vi "Acceleration Move Test.vi"() -> ()   [LabVIEW 2019]
uses:
  <vilib>/rvi/interface/nirviMethod/nirviMethod.xnode
  <vilib>/FPGAPlugInAG/Dynamic/niLvFpga_Abort_Dynamic.vi
  <vilib>/FPGAPlugInAG/Dynamic/niLvFpga_Run_Dynamic.vi
  <vilib>/rvi/interface/nirviReadWriteControl/nirviReadWriteControl.xnode
  NiFpgaLv.dll
  <vilib>/Utility/error.llb/Error Cluster From Error Code.vi
  <vilib>/rvi/interface/Simulation/niFpgaSimulationCallBeginRW.vi
  <vilib>/rvi/errors/niLvFpgaAdjustHostInterfaceError.vi
  <vilib>/platform/TimedLoop/XDataNode/XDataNode.xnode
  <vilib>/Platform/TimedLoop/XDataNode/timing_clust.ctl
  <vilib>/Platform/TimedLoop/XDataNode/XDNodeRunTimeDep.lvlib
  <vilib>/Platform/TimedLoop/XDataNode/wakeup.ctl
  <vilib>/Platform/TimedLoop/XDataNode/nitl_modes.ctl
  <vilib>/rvi/interface/nirviOpenFPGA/nirviOpenFPGA.xnode
  <vilib>/Analysis/NI_AALPro.lvlib
  <vilib>/Instr/_visa.llb/VISA Configure Serial Port (Instr).vi
panel:
  out "實際角度Chart":cluster{"X":dbl, "Y":dbl}(graph)={"X"=-3.299667554384925, "Y"=3.520332445615068} caption="Waveform Chart - dark"
  out "實際角度":cluster{"X":dbl, "Y":dbl, "AccZ":dbl}
  out "Gyro Acceleration Graph":cluster{i32[], "Ideal Acc":dbl[]}[](graph)
  in  "VISA resource name":refnum<visa-resource-name>="COM2"
  out "陀螺儀推算軸長L3":dbl
  out "陀螺儀推算軸長L2":dbl
  out "陀螺儀推算軸長L1":dbl
  out "Axis 3 Real Acceleration Graph":cluster{i32[], "Ideal Acc":dbl[]}[](graph)
  out "Axis 2 Real Acceleration Graph":cluster{i32[], "Ideal Acc":dbl[]}[](graph)
  out "Axis 3 Real Velocity Graph":cluster{i32[], "Ideal Velocity":dbl[]}[](graph)
  out "Axis 2 Real Velocity Graph":cluster{i32[], "Ideal Velocity":dbl[]}[](graph)
  out "Axis 1 Real Acceleration Graph":cluster{i32[], "dX/dt":dbl[]}[](graph)
  out "Axis 1 Real Velocity Graph":cluster{i32[], "Ideal Velocity":dbl[]}[](graph)
  out "Axis 1":cluster{i32[], "Ideal Move":dbl[]}[](graph)
  out "Axis 3":cluster{i32[], "Ideal Move":dbl[]}[](graph)
  out "Axis 2":cluster{i32[], "Ideal Move":dbl[]}[](graph)
  in  "Period":i64=10
  in  "stop":bool
  out "time loop error":errorcluster
  out "Axis 1 速率 (1mm/s)":dbl
  out "Real Period":u32
  out "沖壓":bool
  out "結束了":bool
  out "Voltage\nOutput":dbl
  out "Voltage\nOutput 2":dbl
  out "Voltage\nOutput 3":dbl
  out "Axis 2 速率 (1mm/s)":dbl
  out "Axis 3 速率 (1mm/s)":dbl
  out "shutdown error":errorcluster
  in  "Tab Control":enum32{"Axis Control"}(tab)
  in  "Axis 1~3 Servo on?":bool
  out "Axis 3 Backward Limit":bool
  out "Axis 3 Backward Limit 2":bool
  out "Axis 2 Backward Limit":bool
  out "Axis 2 Backward Limit 2":bool
  in  "Axis 3 Alarm Reset":bool
  in  "Axis 2 Alarm Reset":bool
  in  "Axis 3 Position Reset":bool
  in  "Axis 2 Position Reset":bool
  in  "Axis 1 Alarm Reset":bool
  in  "Axis 1 Position Reset":bool
  in  "Axis 3 Speed":fxp<+/-,64,32>
  in  "Axis 2 Speed":fxp<+/-,64,32>
  out "Axis 3 Encoder Position (Counts)":i32
  out "Axis 2 Encoder Position (Counts)":i32
  out "Axis 1 Encoder Position (Counts)":i32
  in  "Axis 1 Spped":fxp<+/-,64,32>
  in  "Axis 2 Servo on?":bool
  in  "Axis 3 Servo on?":bool
  in  "Axis 1 Servo on?":bool
  out "Axis 1 Forward Limit":bool
  out "Axis 1 Backward Limit":bool
  out "Timed Out?":bool
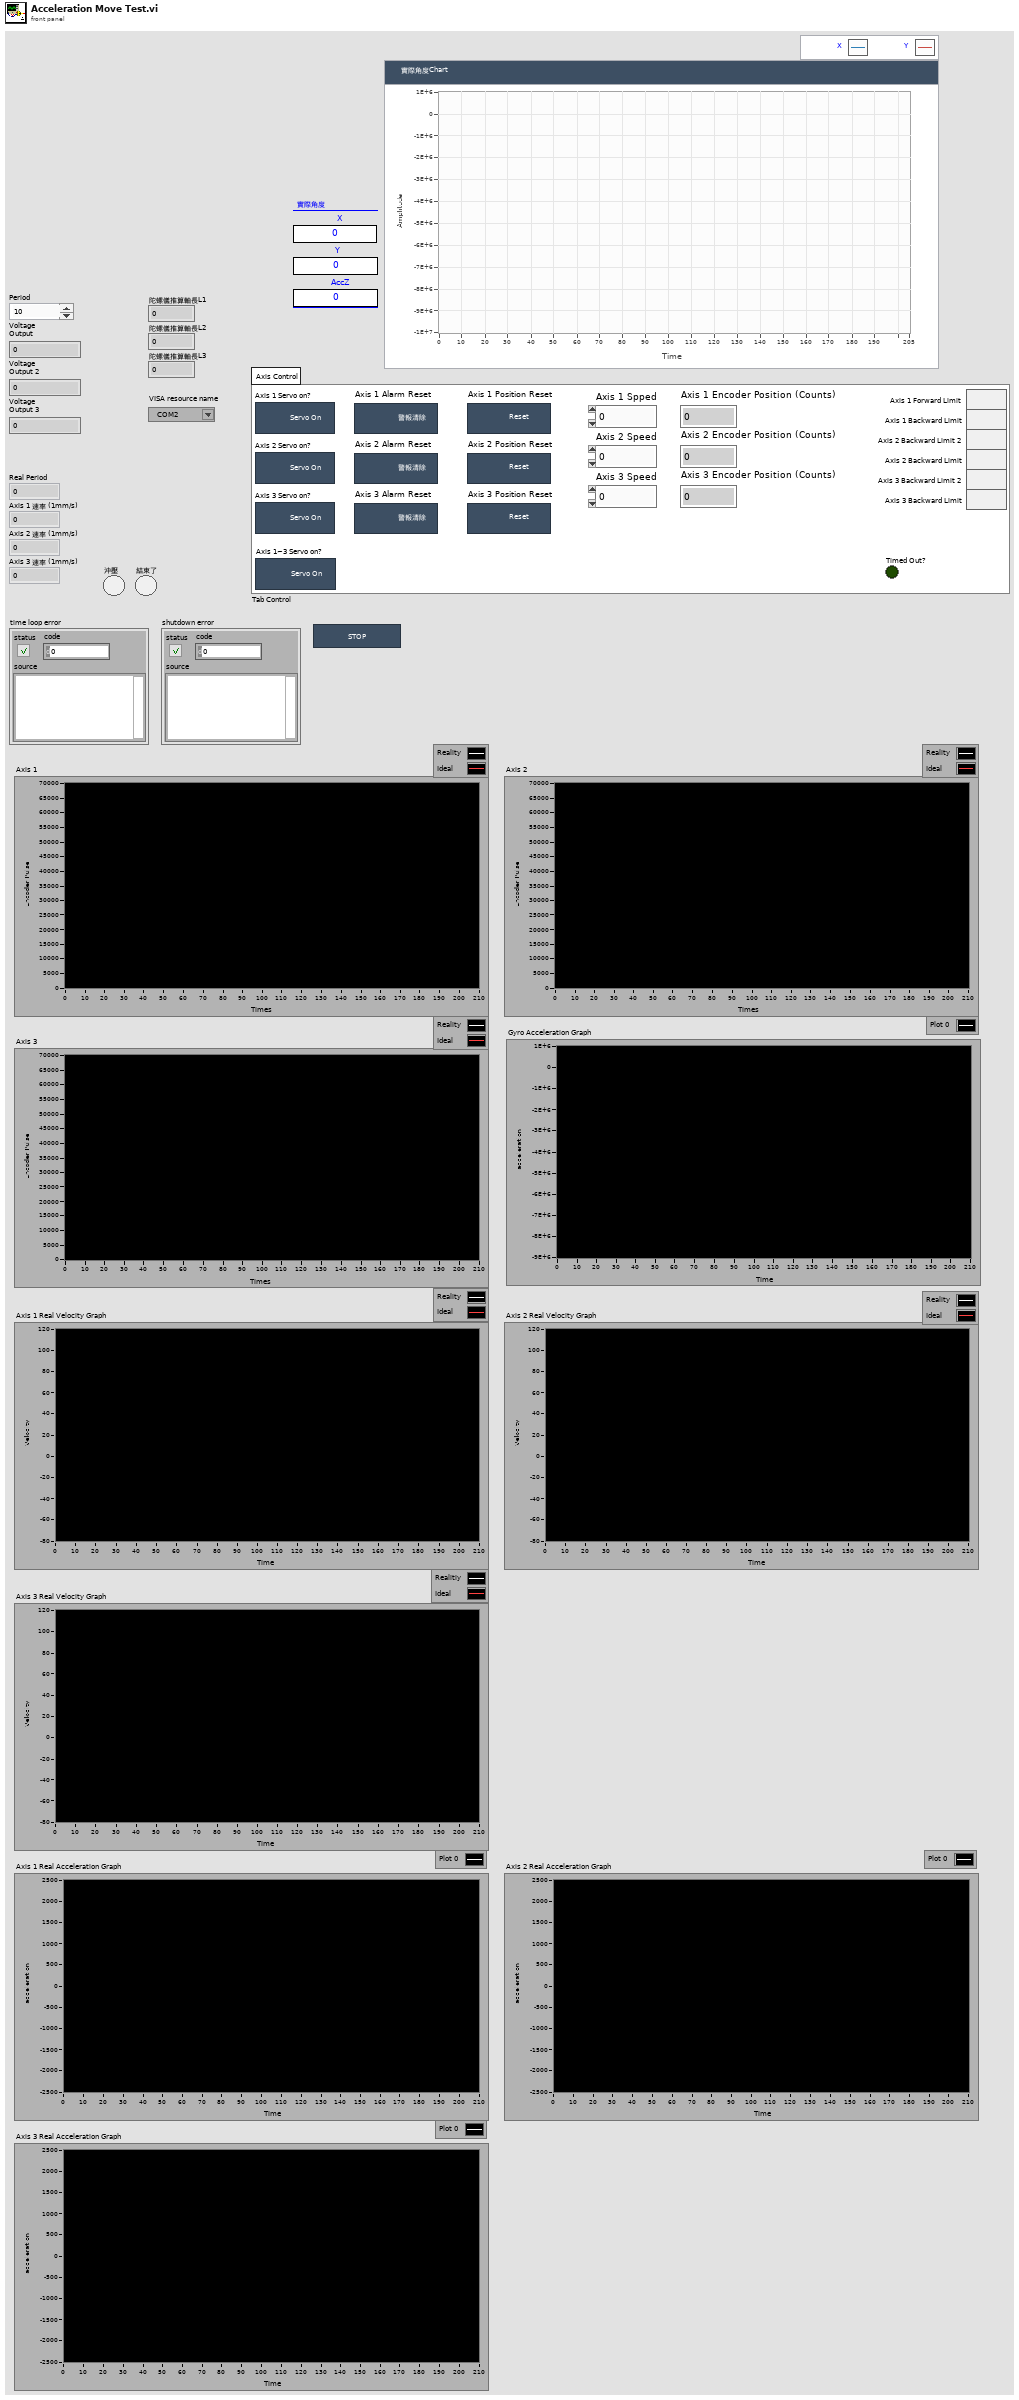
[diagram p1: front panel]
types:
  T1 = enum16{"open", "replace", "create", "open or create", "replace or create", "replace or create with confirmation"}
  T2 = cluster{"Acceleration 1":dbl, "Acceleration 2":dbl, "Acceleration 3":dbl, "Acceleration 4":dbl, "Acceleration 5":dbl, "Acceleration 6":dbl, "Acceleration 7":dbl, "Acceleration 8":dbl}
  T3 = cluster{"Time 1":dbl, "Time 2":dbl, "Time 3":dbl, "Time 4":dbl, "Time 5":dbl, "Time 6":dbl, "Time 7":dbl, "Time 8":dbl}
  T4 = typedef "XDNodeRunTimeDep.lvlib/timing_clust.ctl" = cluster{"Expected End [f-1]":u64, "Actual End [f-1]":u64, "Finished Late? [f-1]":bool, "Expected End [i-1]":u64, "Actual End [i-1]":u64, "Finished Late? [i-1]":bool, "Expected Start [i]":u64, "Actual Start [i]":u64, "Expected Start [f]":u64, "Actual Start [f]":u64, "Source Name":string, "Structure Name":string, "Period":i64, "Deadline":i64, "Offset":i64, "Start":i64, "Priority":i32, "Timeout":i32, "Mode":T5, "Wakeup Reason":T6, "Error":errorcluster, "Source Type":string, "Secondary Source Type":string, "Global End Time":u64, "Global Start Time":u64, "Frame Duration":u64, "Iteration Duration":u64, "Assigned CPU":i32, "I/O Scan Engine Mode":u32}
  T5 = typedef "XDNodeRunTimeDep.lvlib/nitl_modes.ctl" = enum32{"No Change", "Process missed periods, maintain original phase", "Discard missed periods, maintain original phase", "Process missed periods, ignore original phase", "Discard missed periods, ignore original phase"}
  T6 = typedef "XDNodeRunTimeDep.lvlib/wakeup.ctl" = enum32{"Normal", "Aborted", "Asynchronous wakeup", "Timing source error", "Timed loop error", "Timeout"}
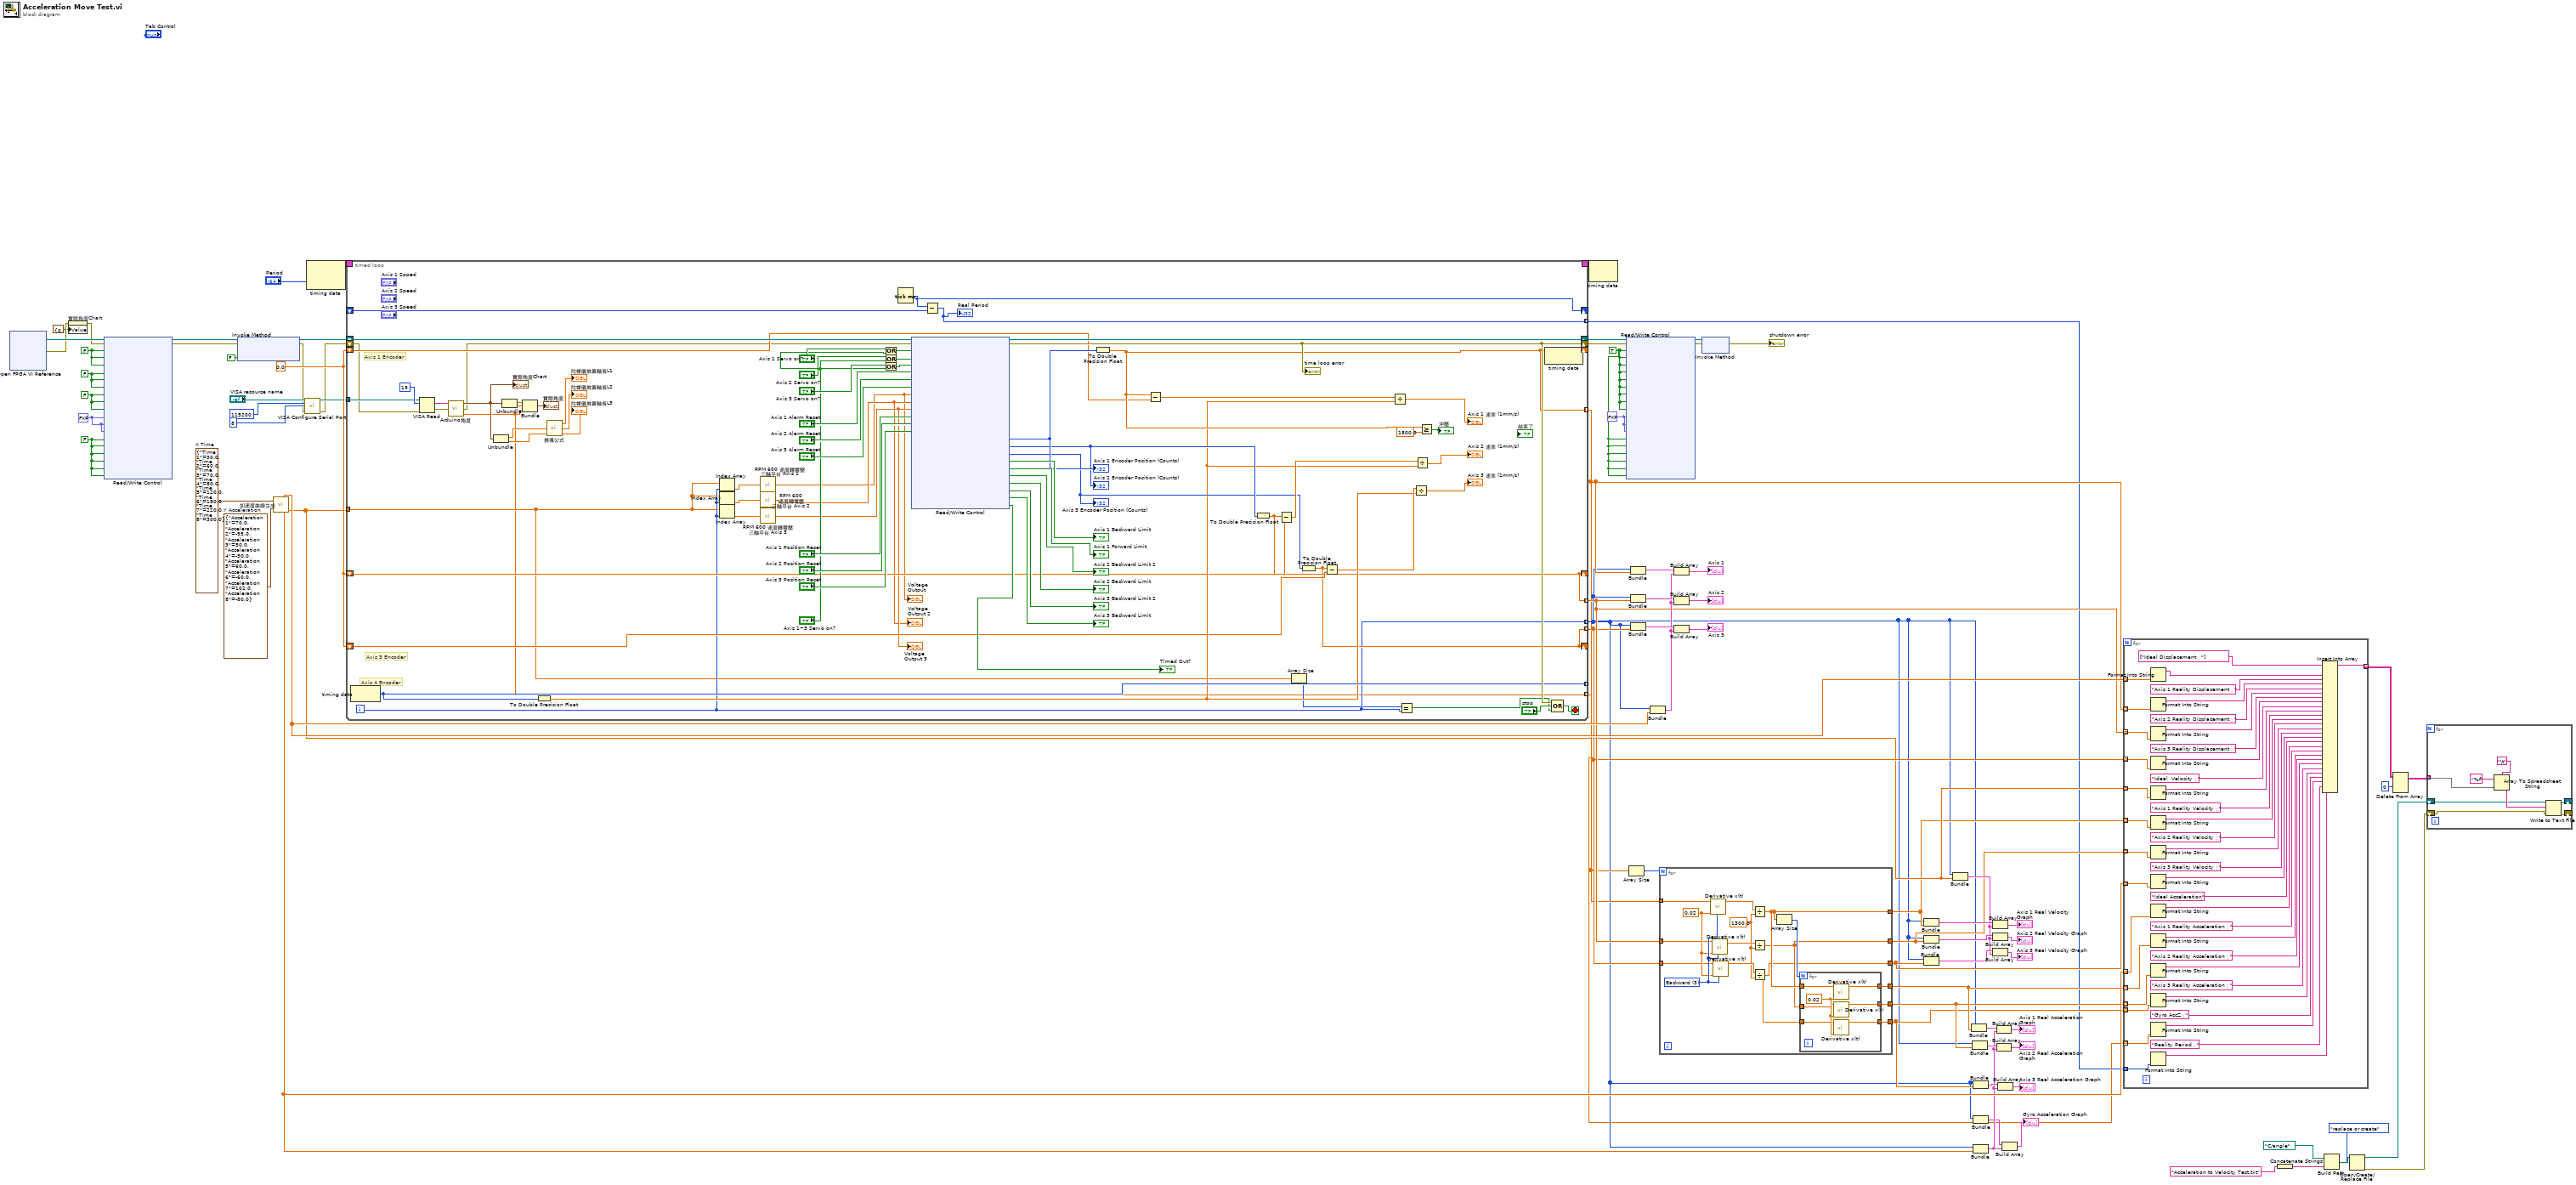
[diagram p0: block diagram]
diagram:
  w58 = T2 {"Acceleration 1"=70.0, "Acceleration 2"=-95.0, "Acceleration 3"=50.0, "Acceleration 4"=-50.0, "Acceleration 5"=60.0, "Acceleration 6"=-60.0, "Acceleration 7"=102.0, "Acceleration 8"=-80.0}  # Y Acceleration
  w60 = T3 {"Time 1"=30.0, "Time 2"=60.0, "Time 3"=70.0, "Time 4"=80.0, "Time 5"=120.0, "Time 6"=180.0, "Time 7"=220.0, "Time 8"=300.0}  # X Time
  w62 = FALSE
  w64 = FALSE
  w70 = 0.0
  w68 = fxp<+,1,1> 0.0
  w67 = TRUE
  w65 = FALSE
  w63 = fxp<+,1,1> 0.0
  w66 = FALSE
  n1 = xnode "Open FPGA VI Reference"() -> ("FPGA VI Reference Out"=w61:refnum<k20>, "error out"=w3:errorcluster)  [unwired: 2 in]
  n2 = property on="實際角度Chart" class="WFChart (strict)"(error in=w3, "Value"=cluster{"X":dbl, "Y":dbl} {"X"=0.0, "Y"=0.0} ("實際角度Chart")) -> (error out=w2:errorcluster)  [unwired: 1 in, 1 out]
  n3 = xnode "Read/Write Control"("FPGA VI Reference In"=w61, "error in"=w2, "Axis 1 Servo on?"=w66, "Axis 2 Servo on?"=w66, "Axis 3 Servo on?"=w66, "Axis 1 Alarm Reset"=w65, "Axis 2 Alarm Reset"=w65, "Axis 3 Alarm Reset"=w65, "Axis 1 Position Reset"=w64, "Axis 2 Position Reset"=w64, "Axis 3 Position Reset"=w64, "Axis 1 Voltage In"=w63, "Axis 2 Voltage In"=w63, "Axis 3 Voltage In"=w63, "Axis 1 Backward Limit"=w62, "Axis 1 Forward Limit"=w62, "Axis 2 Forward Limit"=w62, "Axis 2 Backward Limit"=w62, "Axis 3 ForWard Limit"=w62, "Axis 3 Backward Limit"=w62) -> ("FPGA VI Reference Out"=w79:refnum<k20>, "error out"=w78:errorcluster)
  n4 = xnode "Invoke Method"("FPGA VI Reference In"=w79, "error in"=w78, "Wait Until Done (F)"=FALSE) -> ("FPGA VI Reference Out"=w76:refnum<k20>, "error out"=w10:errorcluster)
  n5 = call "加速度曲線生成.vi"("X Time"=w60, "Y Velocity"=w58) -> ("Ideal Move"=w36:dbl[], "Ideal Acc"=w19:dbl[], "Ideal Velocity"=w32:dbl[])  [unwired: 3 out]
  n6 = call-poly "VISA Configure Serial Port"("VISA resource name"="VISA resource name", "baud rate (9600)"=u32 115200, "data bits (8)"=u16 8, "error in (no error)"=w10) -> ("VISA resource name out"=w11:refnum<visa-resource-name>, "error out"=w9:errorcluster)  [unwired: 10 in]
  n7 = node-c288("Period") -> (w81:T4)  [unwired: 1 in]
  n8 = timed-loop {
    shift-right: [w153] -> w72
    shift-left: w76 -> [w152]
    shift-right: [w120] -> w73
    shift-left: w9 -> [w84]
    timing: w81 -> [_]
    timing-out: [_] -> w80
    shift-right: [w115] -> _
    shift-left: w70 -> [w114]
    tunnel: [w119] -> _ mode=indexing
    shift-right: [w149] -> _
    shift-left: _ -> [w150]
    tunnel: [w109] -> w15 mode=indexing
    shift-right: [w108] -> _
    shift-left: w70 -> [w111]
    shift-right: [w107] -> _
    shift-left: w70 -> [w112]
    tunnel: [w106] -> w7 mode=indexing
    tunnel: [w115] -> w33 mode=indexing
    tunnel: [w108] -> w35 mode=indexing
    tunnel: [w107] -> w34 mode=indexing
    tunnel: w32 -> [w98]
    tunnel: w11 -> [w85]
    tunnel: [w82] -> w4 mode=indexing
    i -> [w106]
    stop <- w151 stop-if-true
    # "Axis 3 Encoder"
    # "Axis 4 Encoder"
    # "Axis 1 Encoder"
    n9 = node-c288() -> (w119:i64)  [unwired: 1 in]
    n10 = VISA Read(VISA resource name=w85, byte count=u32 19, error in (no error)=w84) -> (read buffer=w88:string, error out=w87:errorcluster)  [unwired: 2 out]
    n11 = call "Arduino角度.vi"("error in"=w87, "read buffer"=w88) -> ("AccZ"=w82:dbl, "error out"=w83:errorcluster, "Waveform Chart"=w94:cluster{dbl, dbl})  [unwired: 1 in]
    "實際角度Chart" <- w94
    n12 = Unbundle(w94) -> (w92:dbl, w93:dbl)
    n13 = Unbundle(w94) -> (w95:dbl, w96:dbl)
    n14 = Bundle(w95, w96, "AccZ"=w82) -> (→"實際角度":cluster{dbl, dbl, "AccZ":dbl})  [unwired: 1 in]
    n15 = To Double Precision Float(number=w119) -> (double precision float=w113:dbl)
    n16 = call "推導公式.vi"("be"=w93, "al"=w92) -> ("L3"=→"陀螺儀推算軸長L3":dbl, "L2"=→"陀螺儀推算軸長L2":dbl, "L1"=→"陀螺儀推算軸長L1":dbl)  [unwired: 1 in]
    n17 = Index Array(array=w98, index=w106) -> (element=w103:dbl)
    n18 = Index Array(array=w98, index=w106) -> (element=w102:dbl)
    n19 = Index Array(array=w98, index=w106) -> (element=w104:dbl)
    n20 = call "RPM 600 速度轉電壓 三軸平台 Axis 1.vi"("Speed (1mm/s)"=w103) -> ("Voltage\nOutput"=w99:dbl)
    "Voltage\nOutput" <- w99
    n21 = call "RPM 600 速度轉電壓 三軸平台 Axis 2.vi"("Speed (1mm/s)"=w102) -> ("Voltage\nOutput"=w100:dbl)
    "Voltage\nOutput 2" <- w100
    n22 = call "RPM 600 速度轉電壓 三軸平台 Axis 3.vi"("Speed (1mm/s)"=w104) -> ("Voltage\nOutput"=w101:dbl)
    "Voltage\nOutput 3" <- w101
    n23 = Or(x="Axis 1 Servo on?", y="Axis 1~3 Servo on?") -> (x .or. y?=w132:bool)
    n24 = Or(x="Axis 2 Servo on?", y="Axis 1~3 Servo on?") -> (x .or. y?=w129:bool)
    n25 = Or(x="Axis 3 Servo on?", y="Axis 1~3 Servo on?") -> (x .or. y?=w127:bool)
    n26 = Tick Count (ms)() -> (millisecond timer value=w149:u32)
    n27 = xnode "Read/Write Control"("FPGA VI Reference In"=w152, "error in"=w83, "Axis 1 Servo on?"=w132, "Axis 2 Servo on?"=w129, "Axis 3 Servo on?"=w127, "Axis 1 Alarm Reset"="Axis 1 Alarm Reset", "Axis 2 Alarm Reset"="Axis 2 Alarm Reset", "Axis 3 Alarm Reset"="Axis 3 Alarm Reset", "Axis 1 Voltage In"=w99, "Axis 2 Voltage In"=w100, "Axis 3 Voltage In"=w101, "Axis 1 Position Reset"="Axis 1 Position Reset", "Axis 2 Position Reset"="Axis 2 Position Reset", "Axis 3 Position Reset"="Axis 3 Position Reset") -> ("FPGA VI Reference Out"=w153:refnum<k20>, "error out"=w120:errorcluster, "Axis 1 Encoder Position (Counts)"=w125:i32, "Axis 2 Encoder Position (Counts)"=w123:i32, "Axis 3 Encoder Position (Counts)"=w122:i32, "Axis 1 Backward Limit"=→"Axis 1 Backward Limit":bool, "Axis 1 Forward Limit"=→"Axis 1 Forward Limit":bool, "Axis 2 Backward Limit"=→"Axis 2 Backward Limit 2":bool, "Axis 2 Forward Limit"=→"Axis 2 Backward Limit":bool, "Axis 3 Backward Limit"=→"Axis 3 Backward Limit 2":bool, "Axis 3 ForWard Limit"=→"Axis 3 Backward Limit":bool, "Timed Out?"=→"Timed Out?":bool)
    "time loop error" <- w120
    "Axis 1 Encoder Position (Counts)" <- w125
    "Axis 2 Encoder Position (Counts)" <- w123
    "Axis 3 Encoder Position (Counts)" <- w122
    n28 = Subtract(x=w149, y=w150) -> (x-y=w109:u32)
    "Real Period" <- w109
    n29 = To Double Precision Float(number=w125) -> (double precision float=w115:dbl)
    n30 = Subtract(x=w115, y=w114) -> (x-y=w154:dbl)
    n31 = To Double Precision Float(number=w123) -> (double precision float=w108:dbl)
    n32 = Subtract(x=w108, y=w111) -> (x-y=w124:dbl)
    n33 = Array Size(array=w98) -> (size(s)=w105:i32)
    n34 = To Double Precision Float(number=w122) -> (double precision float=w107:dbl)
    n35 = Subtract(x=w107, y=w112) -> (x-y=w121:dbl)
    n36 = Divide(x=w154, y=w113) -> (x/y=→"Axis 1 速率 (1mm/s)":dbl)
    n37 = Equal?(x=w105, y=w106) -> (x = y?=w110:bool)
    n38 = Divide(x=w121, y=w113) -> (x/y=→"Axis 3 速率 (1mm/s)":dbl)
    n39 = Divide(x=w124, y=w113) -> (x/y=→"Axis 2 速率 (1mm/s)":dbl)
    n40 = Greater Or Equal?(x=w115, y=1800.0) -> (x >= y?=→"沖壓":bool)
    n41 = node-c288() -> ()  [unwired: 1 in, 1 out]
    n42 = Compound Arithmetic op=OR(w120, "stop", w110) -> (w151:bool)
  }
  n43 = node-c288(w80) -> ()  [unwired: 1 out]
  n44 = xnode "Read/Write Control"("FPGA VI Reference In"=w72, "error in"=w73, "Axis 1 Servo on?"=w67, "Axis 2 Servo on?"=w67, "Axis 3 Servo on?"=w67, "Axis 1 Alarm Reset"=w67, "Axis 2 Alarm Reset"=w67, "Axis 3 Alarm Reset"=w67, "Axis 1 Position Reset"=w67, "Axis 2 Position Reset"=w67, "Axis 3 Position Reset"=w67, "Axis 1 Voltage In"=w68, "Axis 2 Voltage In"=w68, "Axis 3 Voltage In"=w68, "Axis 1 Backward Limit"=w67, "Axis 1 Forward Limit"=w67, "Axis 2 Forward Limit"=w67, "Axis 2 Backward Limit"=w67, "Axis 3 ForWard Limit"=w67, "Axis 3 Backward Limit"=w67) -> ("FPGA VI Reference Out"=w75:refnum<k20>, "error out"=w74:errorcluster)
  n45 = Array Size(array=w33) -> (size(s)=w59:i32)
  n46 = Bundle(w7, w33) -> (w50:cluster{i32[], dbl[]})  [unwired: 1 in]
  n47 = Bundle(w7, w35) -> (w49:cluster{i32[], dbl[]})  [unwired: 1 in]
  n48 = Bundle(w7, w34) -> (w48:cluster{i32[], dbl[]})  [unwired: 1 in]
  n49 = Bundle(w7, "Ideal Move"=w36) -> (w47:cluster{i32[], "Ideal Move":dbl[]})  [unwired: 1 in]
  n50 = for {
    N: w59 -> [_]
    tunnel: w33 -> [w173]
    tunnel: [w171] -> w31
    tunnel: [w169] -> w18
    tunnel: w35 -> [w166]
    tunnel: w34 -> [w165]
    tunnel: [w164] -> w17
    tunnel: [w163] -> w16
    tunnel: [w159] -> w30
    tunnel: [w158] -> w29
    w168 = u16 3 items=["2nd Order Central", "4th Order Central", "Forward", "Backward"] ("method")
    w160 = 1300.0 ("dt")
    w167 = 0.02 ("dt")
    n51 = call <vilib>:"Derivative x(t).vi"("method"=w168, "dt"=w167, "X"=w173) -> ("dX/dt"=w172:dbl[])  [unwired: 7 in, 1 out]
    n52 = call <vilib>:"Derivative x(t).vi"("method"=w168, "dt"=w167, "X"=w166) -> ("dX/dt"=w162:dbl[])  [unwired: 7 in, 1 out]
    n53 = call <vilib>:"Derivative x(t).vi"("method"=w168, "dt"=w167, "X"=w165) -> ("dX/dt"=w161:dbl[])  [unwired: 7 in, 1 out]
    n54 = Divide(x=w172, y=w160) -> (x/y=w171:dbl[])
    n55 = Divide(x=w162, y=w160) -> (x/y=w159:dbl[])
    n56 = Divide(x=w161, y=w160) -> (x/y=w158:dbl[])
    n57 = Array Size(array=w171) -> (size(s)=w170:i32)
    n58 = for {
      N: w170 -> [_]
      tunnel: w171 -> [w179]
      tunnel: [w180] -> w169
      tunnel: w159 -> [w177]
      tunnel: w158 -> [w176]
      tunnel: [w175] -> w164
      tunnel: [w174] -> w163
      w178 = 0.02 ("dt")
      n59 = call <vilib>:"Derivative x(t).vi"("dt"=w178, "X"=w179) -> ("dX/dt"=w180:dbl[])  [unwired: 8 in, 1 out]
      n60 = call <vilib>:"Derivative x(t).vi"("dt"=w178, "X"=w177) -> ("dX/dt"=w175:dbl[])  [unwired: 8 in, 1 out]
      n61 = call <vilib>:"Derivative x(t).vi"("dt"=w178, "X"=w176) -> ("dX/dt"=w174:dbl[])  [unwired: 8 in, 1 out]
    }
  }
  n62 = Build Array(w50, w47) -> (→"Axis 1":cluster{i32[], "Ideal Move":dbl[]}[])
  n63 = Build Array(w49, w47) -> (→"Axis 2":cluster{i32[], "Ideal Move":dbl[]}[])
  n64 = Build Array(w48, w47) -> (→"Axis 3":cluster{i32[], "Ideal Move":dbl[]}[])
  n65 = xnode "Invoke Method"("FPGA VI Reference In"=w75, "error in"=w74) -> ("error out"=→"shutdown error":errorcluster)  [unwired: 1 out]
  n66 = Bundle(w7, w31) -> (w57:cluster{i32[], dbl[]})  [unwired: 1 in]
  n67 = Bundle(w7, w30) -> (w56:cluster{i32[], dbl[]})  [unwired: 1 in]
  n68 = Bundle(w7, w29) -> (w55:cluster{i32[], dbl[]})  [unwired: 1 in]
  n69 = Bundle(w7, "Ideal Velocity"=w32) -> (w51:cluster{i32[], "Ideal Velocity":dbl[]})  [unwired: 1 in]
  n70 = Bundle(w7, "dX/dt"=w18) -> (w24:cluster{i32[], "dX/dt":dbl[]})  [unwired: 1 in]
  n71 = Bundle(w7, "dX/dt"=w17) -> (w23:cluster{i32[], "dX/dt":dbl[]})  [unwired: 1 in]
  n72 = Bundle(w7, "dX/dt"=w16) -> (w22:cluster{i32[], "dX/dt":dbl[]})  [unwired: 1 in]
  n73 = Bundle(w7, "Ideal Acc"=w19) -> (w8:cluster{i32[], "Ideal Acc":dbl[]})  [unwired: 1 in]
  n74 = Bundle(w7, w4) -> (w6:cluster{i32[], dbl[]})  [unwired: 1 in]
  n75 = Build Array(w57, w51) -> (→"Axis 1 Real Velocity Graph":cluster{i32[], "Ideal Velocity":dbl[]}[])
  n76 = Build Array(w56, w51) -> (→"Axis 2 Real Velocity Graph":cluster{i32[], "Ideal Velocity":dbl[]}[])
  n77 = Build Array(w55, w51) -> (→"Axis 3 Real Velocity Graph":cluster{i32[], "Ideal Velocity":dbl[]}[])
  n78 = Build Array(w24, w8) -> (→"Axis 1 Real Acceleration Graph":cluster{i32[], "Ideal Acc":dbl[]}[])
  n79 = Build Array(w23, w8) -> (→"Axis 2 Real Acceleration Graph":cluster{i32[], "Ideal Acc":dbl[]}[])
  n80 = Build Array(w22, w8) -> (→"Axis 3 Real Acceleration Graph":cluster{i32[], "Ideal Acc":dbl[]}[])
  n81 = Build Array(w6, w8) -> (→"Gyro Acceleration Graph":cluster{i32[], "Ideal Acc":dbl[]}[])
  n82 = for {
    tunnel: [w222] -> w28 mode=indexing
    tunnel: w36 -> [w219] mode=indexing
    tunnel: w33 -> [w218] mode=indexing
    tunnel: w35 -> [w204] mode=indexing
    tunnel: w34 -> [w203] mode=indexing
    tunnel: w32 -> [w202] mode=indexing
    tunnel: w31 -> [w201] mode=indexing
    tunnel: w30 -> [w200] mode=indexing
    tunnel: w29 -> [w199] mode=indexing
    tunnel: w19 -> [w198] mode=indexing
    tunnel: w18 -> [w189] mode=indexing
    tunnel: w17 -> [w188] mode=indexing
    tunnel: w16 -> [w187] mode=indexing
    tunnel: w15 -> [w186] mode=indexing
    tunnel: w4 -> [w185] mode=indexing
    n83 = Format Into String(w219) -> (resulting string=w221:string)  [unwired: 3 in, 1 out]
    n84 = Format Into String(w218) -> (resulting string=w217:string)  [unwired: 3 in, 1 out]
    n85 = Format Into String(w204) -> (resulting string=w215:string)  [unwired: 3 in, 1 out]
    n86 = Format Into String(w203) -> (resulting string=w213:string)  [unwired: 3 in, 1 out]
    n87 = Format Into String(w202) -> (resulting string=w211:string)  [unwired: 3 in, 1 out]
    n88 = Format Into String(w201) -> (resulting string=w209:string)  [unwired: 3 in, 1 out]
    n89 = Format Into String(w200) -> (resulting string=w207:string)  [unwired: 3 in, 1 out]
    n90 = Format Into String(w199) -> (resulting string=w205:string)  [unwired: 3 in, 1 out]
    n91 = Format Into String(w198) -> (resulting string=w196:string)  [unwired: 3 in, 1 out]
    n92 = Format Into String(w189) -> (resulting string=w194:string)  [unwired: 3 in, 1 out]
    n93 = Format Into String(w188) -> (resulting string=w192:string)  [unwired: 3 in, 1 out]
    n94 = Format Into String(w187) -> (resulting string=w190:string)  [unwired: 3 in, 1 out]
    n95 = Format Into String(w185) -> (resulting string=w183:string)  [unwired: 3 in, 1 out]
    n96 = Format Into String(w186) -> (resulting string=w181:string)  [unwired: 3 in, 1 out]
    n97 = Insert Into Array(array=string[] ["Ideal Displacement："], new element #1=w221, new element #2="Axis 1 Reality Displacement：", new element #3=w217, new element #4="Axis 2 Reality Displacement：", new element #5=w215, new element #6="Axis 3 Reality Displacement：", new element #7=w213, new element #8="Ideal  Velocity：", new element #9=w211, new element #10="Axis 1 Reality Velocity：", new element #11=w209, new element #12="Axis 2 Reality Velocity：", new element #13=w207, new element #14="Axis 3 Reality Velocity：", new element #15=w205, new element #16="Ideal Acceleration", new element #17=w196, new element #18="Axis 1 Reality Acceleration：", new element #19=w194, new element #20="Axis 2 Reality Acceleration：", new element #21=w192, new element #22="Axis 3 Reality Acceleration：", new element #23=w190, new element #24="Gyro AccZ：", new element #25=w183, new element #26="Reality Period：", new element #27=w181) -> (w222:string[])  [unwired: 1 in]
  }
  n98 = Concatenate Strings("Acceleration to Velocity Test.txt" ("element")) -> (w42:string)
  n99 = Build Path(base path=path "C:/angle", name or relative path=w42) -> (appended path=w43:path)
  n100 = Open/Create/Replace File(file path (use dialog)=w43, operation (0:open)=T1."replace or create") -> (refnum out=w27:refnum<file>, error out=w26:errorcluster)  [unwired: 4 in, 1 out]
  n101 = Delete From Array(array=w28, index (row)=0) -> (array with subset deleted=w38:string[][])  [unwired: 2 in, 1 out]
  n102 = for {
    shift-right: [w225] -> _
    shift-left: w27 -> [w228]
    shift-right: [w226] -> _
    shift-left: w26 -> [w227]
    tunnel: w38 -> [w224] mode=indexing
    n103 = Array To Spreadsheet String(delimiter (Tab)="\t", array=w224, 3:"%f" ("format string")) -> (spreadsheet string=w229:string)
    n104 = Write to Text File(file (use dialog)=w228, text=w229, error in=w227) -> (refnum out=w225:refnum<file>, error out=w226:errorcluster)  [unwired: 1 in, 1 out]
  }
